vi "parse_range_roslv.vi"(4 "error in":errorcluster, 7 "msg in":string) -> (0 "error out":errorcluster, 1 "Header":T1, 2 "Range Data":T2, 3 "msg out":string)   [LabVIEW 2014]
doc: "Parses a message into a range"
uses:
  std_msgs/subs/parse_u8_scalar_roslv.vi
  std_msgs/subs/parse_float32_scalar_roslv.vi
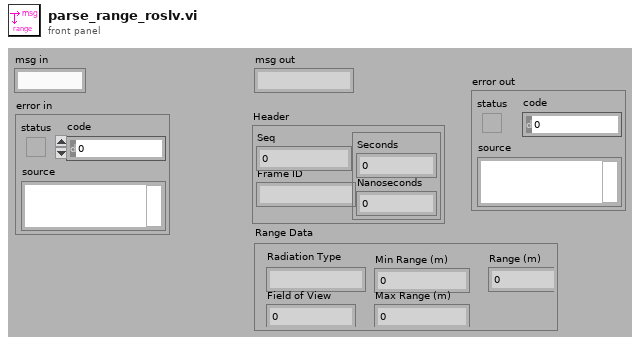
[diagram p1: front panel]
types:
  T1 = cluster{"Seq":u32, "Frame ID":string, cluster{"Seconds":i32, "Nanoseconds":i32}}
  T2 = cluster{"Radiation Type":string, "Field of View":sgl, "Min Range (m)":sgl, "Max Range (m)":sgl, "Range (m)":sgl}
  T3 = cluster{"Seq":u32, "Frame ID":string, "Timestamp":cluster{"Seconds":i32, "Nanoseconds":i32}}
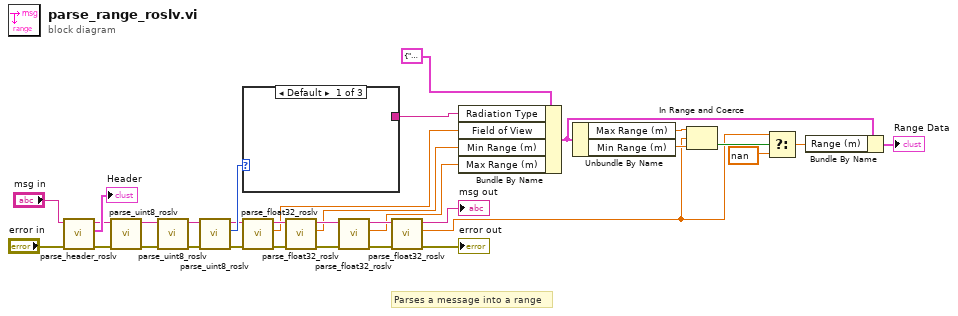
[diagram p0: block diagram]
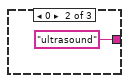
[diagram p2: hidden frame]
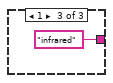
[diagram p3: hidden frame]
diagram:
  # "Parses a message into a range"
  n1 = call "parse_header_roslv.vi"("error in"="error in", "msg in"="msg in") -> ("error out"=w4:errorcluster, "Header"=→"Header":T3, "msg out"=w3:string)  [unwired: 3 in]
  n2 = call-poly "parse_uint8_roslv.vi"("error in"=w4, "msg in"=w3) -> ("error out"=w8:errorcluster, "msg out"=w7:string)  [unwired: 3 in, 1 out]
  n3 = call-poly "parse_uint8_roslv.vi"("error in"=w8, "msg in"=w7) -> ("error out"=w2:errorcluster, "msg out"=w1:string)  [unwired: 3 in, 1 out]
  n4 = call-poly "parse_uint8_roslv.vi"("error in"=w2, "msg in"=w1) -> ("error out"=w28:errorcluster, "number"=w31:u8, "msg out"=w29:string)  [unwired: 3 in]
  n5 = case shown="Default" w31 {
    tunnel: [_ "ultrasound" "infrared"] -> w30
    frame Default {
    }
    frame 0 {
    }
    frame 1 {
    }
  }
  n6 = call-poly "parse_float32_roslv.vi"("error in"=w28, "msg in"=w29) -> ("error out"=w26:errorcluster, "number"=w19:sgl, "msg out"=w27:string)  [unwired: 3 in]
  n7 = call-poly "parse_float32_roslv.vi"("error in"=w26, "msg in"=w27) -> ("error out"=w25:errorcluster, "number"=w18:sgl, "msg out"=w24:string)  [unwired: 3 in]
  n8 = call-poly "parse_float32_roslv.vi"("error in"=w25, "msg in"=w24) -> ("error out"=w22:errorcluster, "number"=w17:sgl, "msg out"=w23:string)  [unwired: 3 in]
  n9 = call-poly "parse_float32_roslv.vi"("error in"=w22, "msg in"=w23) -> ("error out"=→"error out":errorcluster, "number"=w9:sgl, "msg out"=→"msg out":string)  [unwired: 3 in]
  n10 = Bundle By Name(cluster=T2 {"Radiation Type"="", "Field of View"=0.0, "Min Range (m)"=0.0, "Max Range (m)"=0.0, "Range (m)"=0.0} ("Range Data"), "Radiation Type"=w30, "Field of View"=w19, "Min Range (m)"=w18, "Max Range (m)"=w17) -> (w11:T2)
  n11 = Unbundle By Name(w11) -> ("Max Range (m)"=w14:sgl, "Min Range (m)"=w15:sgl)
  n12 = In Range and Coerce(upper limit=w14, x=w9, lower limit=w15) -> (In Range?=w12:bool)  [unwired: 1 out]
  n13 = Select(t=w9, s=w12, f=sgl nan) -> (s? t:f=w16:sgl)
  n14 = Bundle By Name(cluster=w11, "Range (m)"=w16) -> (→"Range Data":T2)
